vi "Main_UI_AutoPaste.vi"(8 "error in (no error)":errorcluster) -> (0 "error out":errorcluster)   [LabVIEW 2019]
uses:
  <vilib>/Utility/miscctls.llb/LVPointTypeDef.ctl
  <vilib>/Utility/miscctls.llb/LVPositionTypeDef.ctl
  Ctrl/tray icon.ctl
  Function/Main UI/Glb/Main_UI Gb.vi
  LLB/Commonly VI.lvlib
panel:
  in  "Tab Control":enum32{"Page 1", "Page 2"}(tab)
  in  "Station Name 3":string="Pick"
  in  "Station Name 2":string="AI"
  in  "Station Name 1":string="Line Scan"
  out "Image 2":T1(plugin-control)
  in  "TrayStatus":u32[][](array[colorbox])
  out "Image":T1(plugin-control)
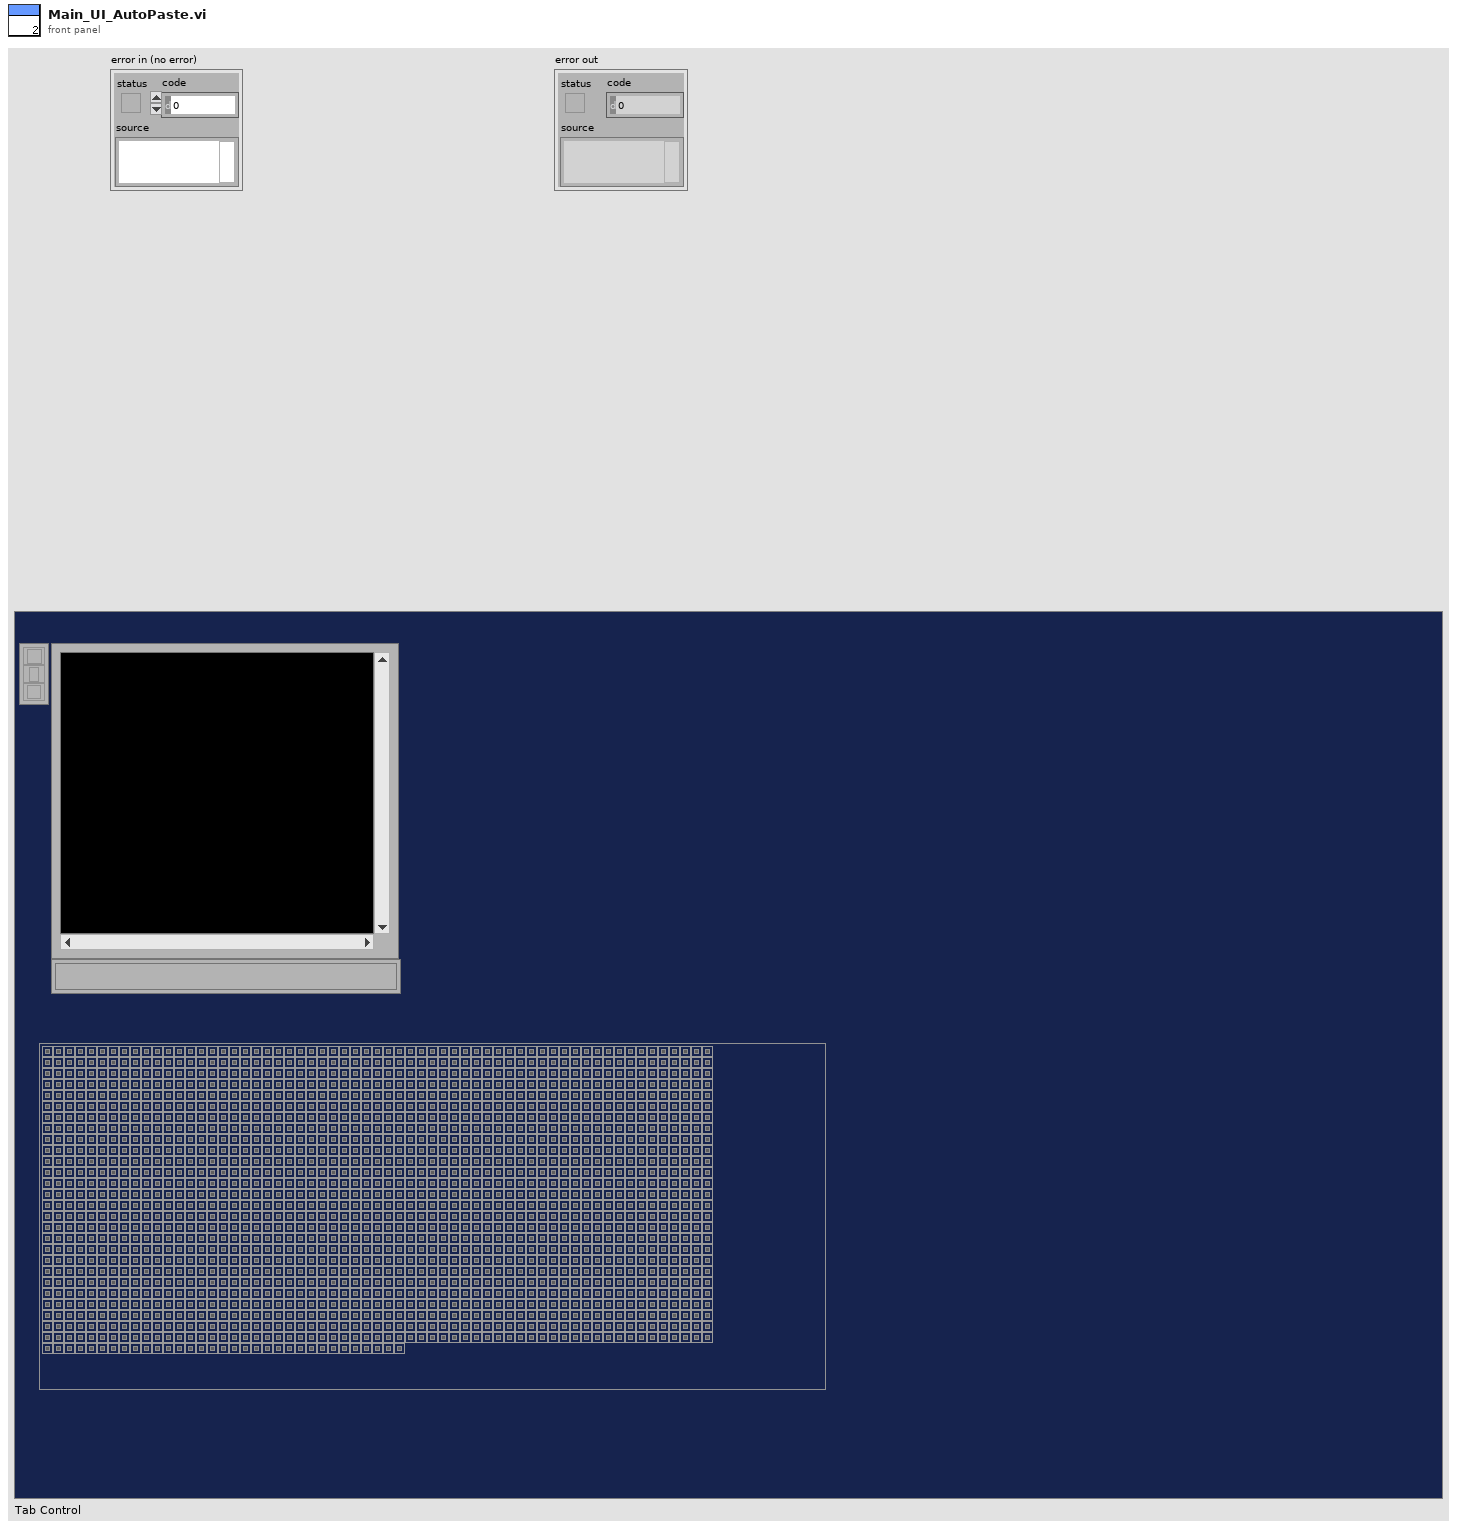
[diagram p1: front panel]
types:
  T1 = typedef "IMAQ Image.ctl" = refnum<image>
  T2 = typedef "LVPositionTypeDef.ctl" = cluster{"Left":i32, "Top":i32}
  T3 = typedef "LVPointTypeDef.ctl" = cluster{"Horizontal":i16, "Vertical":i16}
  T4 = typedef "tray icon.ctl" = u16
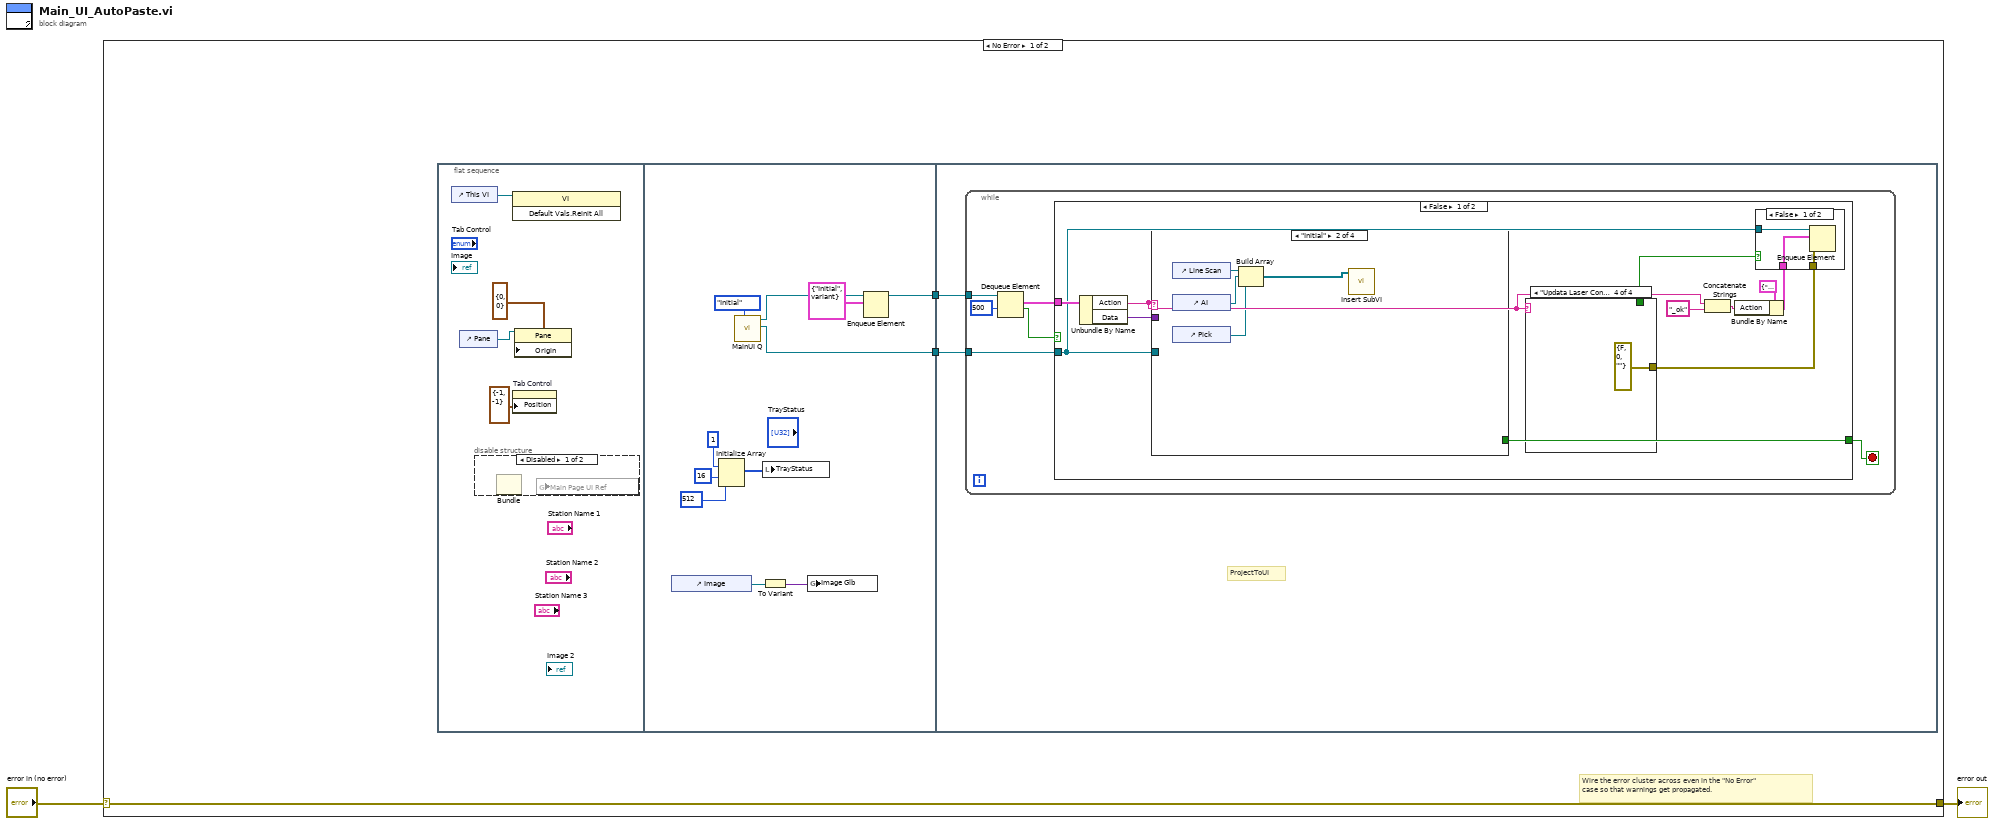
[diagram p0: block diagram]
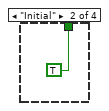
[diagram p5: hidden frame]
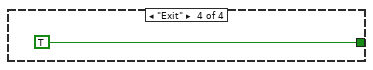
[diagram p9: hidden frame]
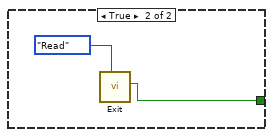
[diagram p10: hidden frame]
diagram:
  n1 = case shown="No Error" "error in (no error)" {
    selector: "error in (no error)" -> [w5 w52]
    tunnel: [w5 w52] -> w1
    frame No Error {
      # "Wire the error cluster across even in the \"No Error\"\ncase so that warnings get propagated."
      n2 = flat-sequence {
        tunnel: [w20] -> w4
        tunnel: [w16] -> w3
        tunnel: w4 -> [w22]
        tunnel: w3 -> [w21]
        frame #0 {
          n3 = control-ref of="This VI"() -> (w6:refnum<vi>)
          n4 = control-ref of="Pane"() -> (w9:refnum<vi>)
          n5 = disable-structure shown="Disabled" {
            frame Disabled {
              n6 = Bundle() -> ()  [unwired: 4 in, 1 out]
              n7 = global read "Main_UI Gb.vi" "Main Page UI Ref"() -> ()  [unwired: 1 in]
            }
            frame Enabled {
            }
          }
          n8 = invoke class="VI" method="Default Vals.Reinit All"(reference=w6) -> ()  [unwired: 2 in, 3 out]
          n9 = property on="Tab Control" class="TabCtl (strict)"("Position"=T2 {"Left"=-1, "Top"=-1}) -> ()  [unwired: 2 in, 2 out]
          n10 = property class="Pane"(reference=w9, "Origin"=T3 {"Horizontal"=0, "Vertical"=0}) -> ()  [unwired: 1 in, 2 out]
        }
        frame #1 {
          n11 = control-ref of="Image"() -> (w15:refnum<vi>)
          n12 = Initialize Array(T4 1 ("Ring"), 16 ("dimension size"), 512 ("dimension size")) -> (w10:T4[][])
          n13 = call "MainUI Q.vi"("Enum"=enum16{"Initial", "read", "release"}."Initial") -> ("UI Response Out"=w16:refnum<queue>, "UI Receive Out"=w17:refnum<queue>)  [unwired: 9 in]
          n14 = local write "TrayStatus"(w10) -> ()
          n15 = To Variant(anything=w15) -> (Variant=w14:variant)
          n16 = global write "Main_UI Gb.vi" "Image Glb"(w14) -> ()
          n17 = Enqueue Element(queue=w17, element=cluster{"Action":string, "Data":variant} {"Action"="Initial", "Data"=variant}) -> (queue out=w20:refnum<queue>)  [unwired: 2 in, 2 out]
        }
        frame #2 {
          # "ProjectToUI"
          n18 = while {
            tunnel: w22 -> [w28]
            tunnel: w21 -> [w26]
            stop <- w25 stop-if-true
            n19 = Dequeue Element(queue=w28, timeout in ms (-1)=500) -> (element=w27:cluster{"Action":string, "Data":variant}, timed out?=w24:bool)  [unwired: 1 in, 2 out]
            n20 = case shown="False" w24 {
              tunnel: w27 -> [w39 _]
              tunnel: w26 -> [w36 _]
              tunnel: [w38 w51] -> w25
              frame False {
                n21 = Unbundle By Name(w39) -> ("Action"=w32:string, "Data"=w37:variant)
                n22 = case shown="\"Initial\"" w32 {
                  tunnel: w36 -> [_ _ _ _]
                  tunnel: [_ _ _ TRUE] -> w38
                  tunnel: w37 -> [_ _ _ _]
                  frame "False", Default {
                  }
                  frame "Initial" {
                    n23 = control-ref of="Line Scan"() -> (w48:refnum<vi>)
                    n24 = control-ref of="AI"() -> (w47:refnum<vi>)
                    n25 = control-ref of="Pick"() -> (w46:refnum<vi>)
                    n26 = Build Array(w48, w47, w46) -> (w45:refnum<vi>[])
                    n27 = call "Insert SubVI.vi"("Sub UI"=w45) -> ()  [unwired: 11 in]
                  }
                  frame "SetSyms" {
                  }
                  frame "Exit" {
                  }
                }
                n28 = case shown="\"Updata Laser Connect\"" w32 {
                  tunnel: [_ _ _ errorcluster {"status"=FALSE, "code"=0, "source"=""} ("error constant")] -> w30
                  tunnel: [_ TRUE _ _] -> w29
                  frame "False", Default {
                  }
                  frame "Initial" {
                  }
                  frame "ProjectToUI" {
                  }
                  frame "Updata Laser Connect" {
                  }
                }
                n29 = Concatenate Strings(w32, "_ok" ("string")) -> (w33:string)
                n30 = Bundle By Name(cluster=cluster{"Action":string, "Data":variant} {"Action"="", "Data"=variant} ("element"), "Action"=w33) -> (w34:cluster{"Action":string, "Data":variant})
                n31 = case shown="False" w29 {
                  tunnel: w36 -> [w42 _]
                  tunnel: w34 -> [w41 _]
                  tunnel: w30 -> [w40 _]
                  frame False {
                    n32 = Enqueue Element(queue=w42, element=w41, error in (no error)=w40) -> ()  [unwired: 1 in, 3 out]
                  }
                  frame True {
                  }
                }
              }
              frame True {
                n33 = call "Exit.vi"("Enum"=enum16{"Initial", "Read", "Write"}."Read") -> ("ExitOut"=w51:bool)  [unwired: 10 in]
              }
            }
          }
        }
      }
    }
    frame Error {
    }
  }
  "error out" <- w1
